vi "UI Header Data.vi"(8 "error in (no error)":errorcluster, 11 "C&C Data In":T1 {"Hardware Configuration"."Reference Distance" format="%.3g"}) -> (0 "error out":errorcluster, 2 "Header String out":string, 3 "C&C Data Out":T1 {"Hardware Configuration"."Reference Distance" format="%.3g"})   [LabVIEW 2018]
uses:
  Settings/Settings.ctl
  Acquisition/Hardware Configuration.ctl
  Logging/Logging Configuration.ctl
  <vilib>/addons/database/Connection.llb/Conn ObjectReference.ctl
  Controls/Location Ring.ctl
  Controls/Time Remaining.ctl
  OSTEP_MySQLdBTools/MySQLTools.lvlib
  Acquisition/Acquisition.lvlib
  <vilib>/addons/database/NI_Database_API.lvlib
  Logging/Logging.lvlib
  Settings/Settings.lvlib
panel:
  # "example output\n\nOperator: Winston Hensley\nLocation: Chesapeake\nStart Time(UTC): 12/19/2017 08:35\nReference Distance(m): 2.227"
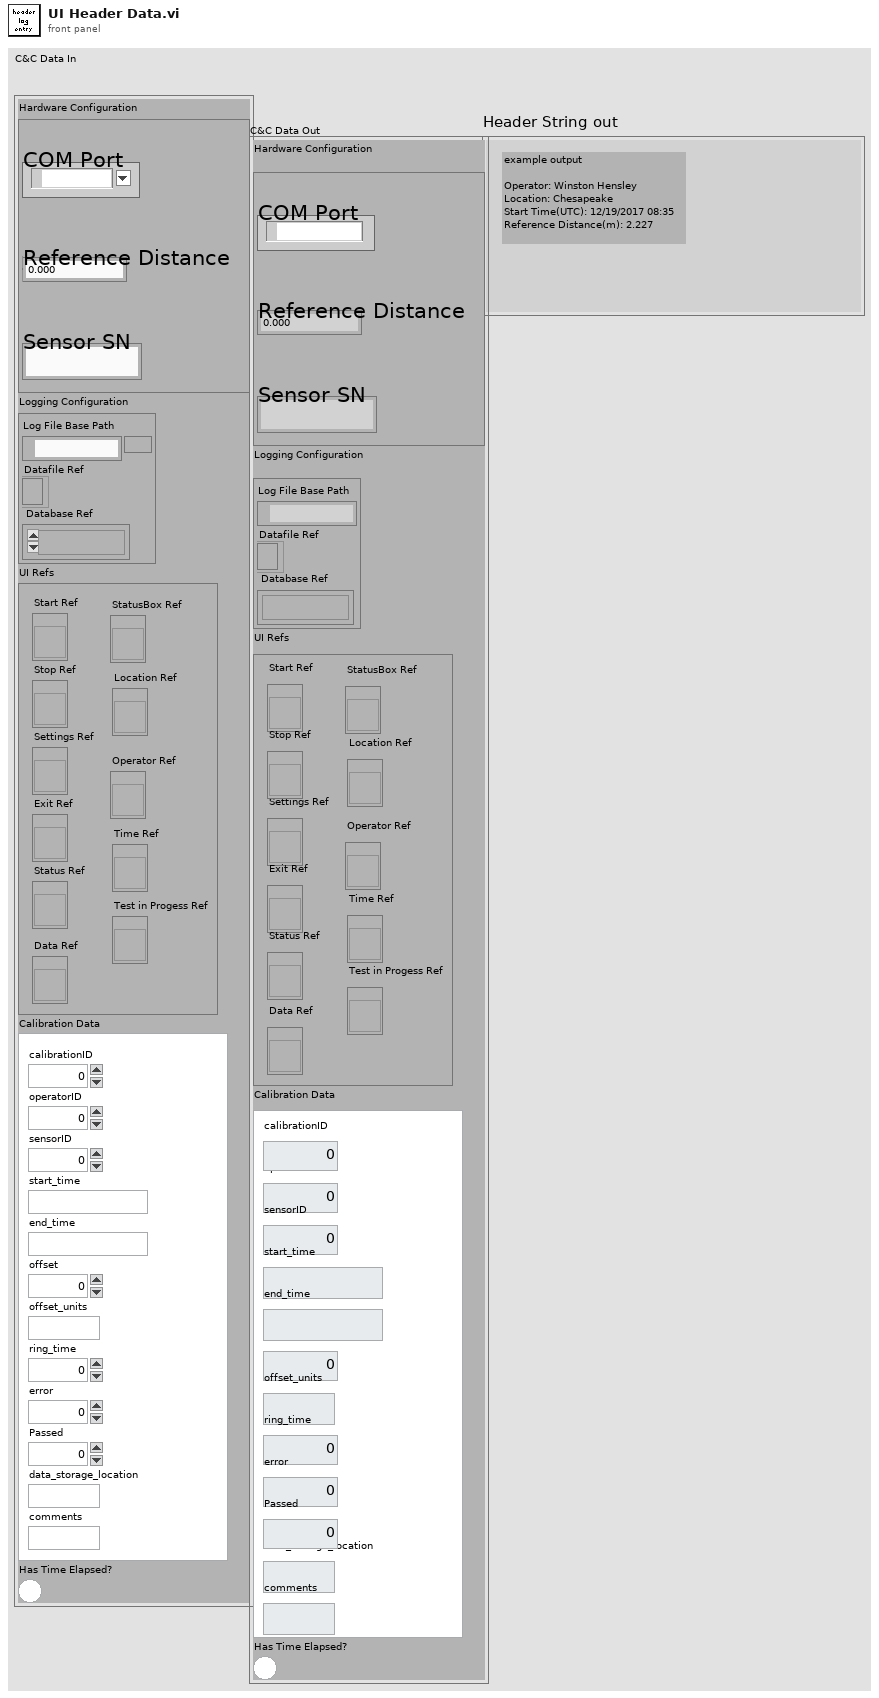
[diagram p1: front panel]
types:
  T1 = typedef "Settings.lvlib/Settings.ctl" = cluster{"Hardware Configuration":T2, "Logging Configuration":T3, "UI Refs":cluster{"Start Ref":refnum<vi>, "Settings Ref":refnum<vi>, "Stop Ref":refnum<vi>, "Exit Ref":refnum<vi>, "Status Ref":refnum<vi>, "Data Ref":refnum<vi>, "StatusBox Ref":refnum<vi>, "Location Ref":refnum<vi>, "Operator Ref":refnum<vi>, "Time Ref":refnum<vi>, "Test in Progess Ref":refnum<vi>}, "Calibration Data":cluster{"calibrationID":u16, "operatorID":u16, "sensorID":u16, "start_time":string, "end_time":string, "offset":dbl, "offset_units":string, "ring_time":dbl, "error":dbl, "Passed":u8, "data_storage_location":string, "comments":string}, "Has Time Elapsed?":bool}
  T2 = typedef "Acquisition.lvlib/Hardware Configuration.ctl" = cluster{"COM Port":refnum<visa-resource-name>, "Reference Distance":dbl, "Sensor SN":string}
  T3 = typedef "Logging.lvlib/Logging Configuration.ctl" = cluster{"Log File Base Path":path, "Datafile Ref":refnum<file>, "Database Ref":T4}
  T4 = typedef "NI_Database_API.lvlib/Conn ObjectReference.ctl" = refnum<k1>
  T5 = cluster{"calibrationID":u16, "operatorID":u16, "sensorID":u16, "start_time":string, "end_time":string, "offset":dbl, "offset_units":string, "ring_time":dbl, "error":dbl, "Passed":u8, "data_storage_location":string, "comments":string}
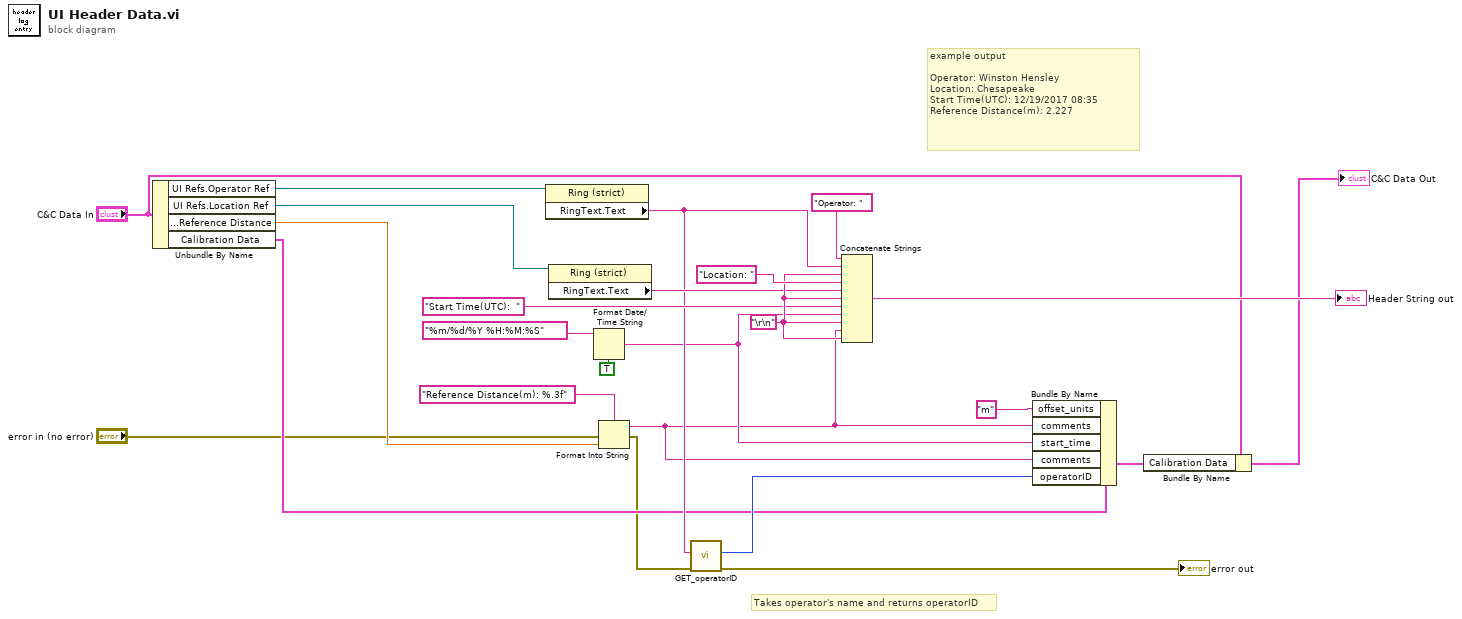
[diagram p0: block diagram]
diagram:
  w19 = "\r\n"
  # "Takes operator's name and returns operatorID"
  # "example output\n\nOperator: Winston Hensley\nLocation: Chesapeake\nStart Time(UTC): 12/19/2017 08:35\nReference Distance(m): 2.227"
  n1 = Unbundle By Name("C&C Data In") -> ("UI Refs.Operator Ref"=w17:refnum<vi>, "UI Refs.Location Ref"=w16:refnum<vi>, "Hardware Configuration.Reference Distance"=w15:dbl, "Calibration Data"=w8:T5)
  n2 = property class="Ring (strict)"(reference=w17) -> ("RingText.Text"=w12:string)  [unwired: 1 in, 2 out]
  n3 = property class="Ring (strict)"(reference=w16) -> ("RingText.Text"=w13:string)  [unwired: 1 in, 2 out]
  n4 = Format Date/Time String(time format string (%c)="%m/%d/%Y %H:%M:%S" ("string"), UTC format=TRUE) -> (date/time string=w9:string)  [unwired: 1 in]
  n5 = Format Into String(format string="Reference Distance(m): %.3f", error in="error in (no error)", w15) -> (resulting string=w5:string, error out=w7:errorcluster)  [unwired: 1 in]
  n6 = call "GET_operatorID.vi"("error in (no error)"=w7, "Operator Full Name"=w12) -> ("error out"=→"error out":errorcluster, "operatorID"=w10:u16)  [unwired: 8 in]
  n7 = Concatenate Strings("Operator: " ("string"), w12, w19, "Location: " ("string"), w13, w19, "Start Time(UTC):  " ("string"), w9, w19, w5, w19) -> (→"Header String out":string)
  n8 = Bundle By Name(cluster=w8, "offset_units"="m" ("string"), "comments"=w5, "start_time"=w9, "comments"=w5, "operatorID"=w10) -> (w3:T5)
  n9 = Bundle By Name(cluster="C&C Data In", "Calibration Data"=w3) -> (→"C&C Data Out":T1)
